vi "Close Error Handles.vi"(8 "error in":errorcluster, 11 "VS Plugin Inline Async API in":refnum<class "VS Plugin Inline Async API.lvclass">) -> (0 "error out":errorcluster, 3 "VS Plugin Inline Async API out":refnum<class "VS Plugin Inline Async API.lvclass">)   [LabVIEW 2024, in "VS Plugin Inline Async API.lvlib" / "VS Plugin Inline Async API.lvclass"]
uses:
  VS Plugin Inline Async API.lvclass
  VS Plugin Inline Async API.lvclass/VS Plugin Inline Async API.ctl
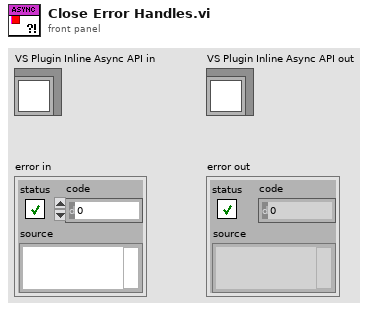
[diagram p1: front panel]
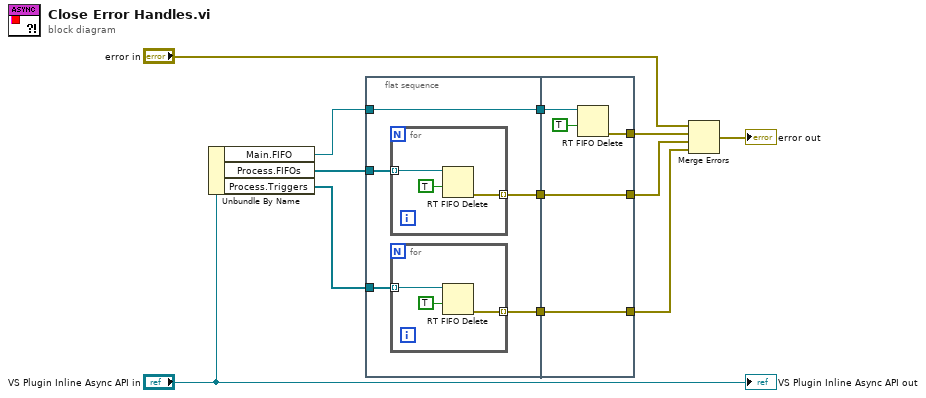
[diagram p0: block diagram]
diagram:
  n1 = Unbundle By Name("VS Plugin Inline Async API in") -> ("Main.FIFO"=w5:refnum<k33>, "Process.FIFOs"=w6:refnum<k33>[], "Process.Triggers"=w3:refnum<k33>[])
  n2 = flat-sequence {
    tunnel: w6 -> [w17]
    tunnel: [w16] -> w9
    tunnel: w5 -> [w16]
    tunnel: [w15] -> w8
    tunnel: w3 -> [w14]
    tunnel: [w13] -> w7
    tunnel: w9 -> [w27]
    tunnel: [w28] -> w12
    tunnel: [w26] -> w4
    tunnel: w8 -> [w26]
    tunnel: w7 -> [w24]
    tunnel: [w24] -> w2
    frame #0 {
      n3 = for {
        tunnel: w17 -> [w22] mode=indexing
        tunnel: [w23] -> w15 mode=indexing
        n4 = RT FIFO Delete(0:w22, 2:TRUE ("force destroy? (F)")) -> (11:w23:errorcluster)  [unwired: 1 in]
      }
      n5 = for {
        tunnel: w14 -> [w19] mode=indexing
        tunnel: [w20] -> w13 mode=indexing
        n6 = RT FIFO Delete(0:w19, 2:TRUE ("force destroy? (F)")) -> (11:w20:errorcluster)  [unwired: 1 in]
      }
    }
    frame #1 {
      n7 = RT FIFO Delete(0:w27, 2:TRUE ("force destroy? (F)")) -> (11:w28:errorcluster)  [unwired: 1 in]
    }
  }
  n8 = Merge Errors("error in", w12, w4, w2) -> (→"error out":errorcluster)
  "VS Plugin Inline Async API out" <- "VS Plugin Inline Async API in"
